vi "Validate Range.vi"(8 "error in (no error)":errorcluster, 11 "Varian Magnet Scan in":refnum<class "Varian Magnet Scan.lvclass">) -> (0 "error out":errorcluster, 3 "Varian Magnet Scan out":refnum<class "Varian Magnet Scan.lvclass">)   [LabVIEW 2009, in "Varian Magnet Scan.lvclass"]
doc: "Coerce the range to be within this Scanner's physical limits."
uses:
  Varian Magnet Scan.lvclass
  Scanner/Scanner.lvclass
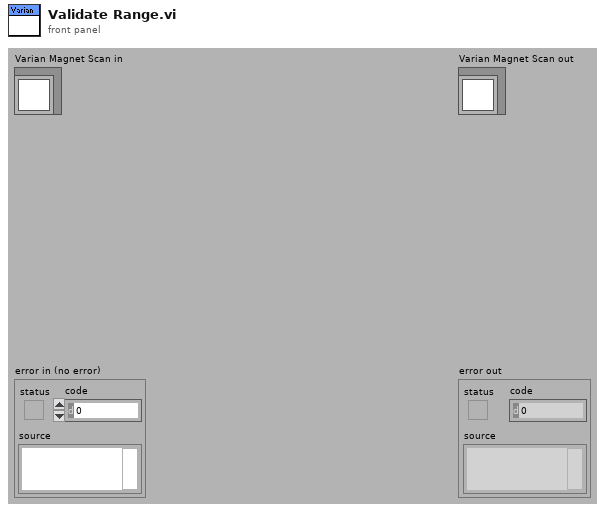
[diagram p1: front panel]
types:
  T1 = typedef "Scanner.lvclass/Range.ctl" = cluster{"xi":dbl, "xf":dbl, "dx":dbl, "Return to...?":bool, "Return to":dbl}
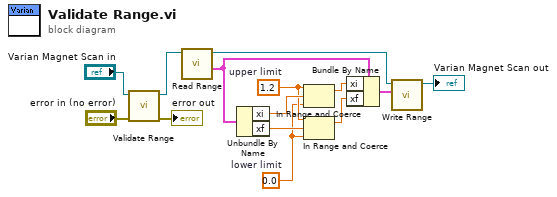
[diagram p0: block diagram]
diagram:
  w8 = 0.0  # lower limit
  w9 = 1.2  # upper limit
  n1 = call-parent "Validate Range.vi"("error in (no error)"="error in (no error)", "Scanner in"="Varian Magnet Scan in") -> ("error out"=→"error out":errorcluster, "Scanner out"=w1:refnum<class "Varian Magnet Scan.lvclass">)  [unwired: 8 in]
  n2 = call-dynamic "Read Range.vi"("Scanner.lvclass in"=w1) -> ("Range"=w6:T1, "Scanner.lvclass out"=w3:refnum<class "Varian Magnet Scan.lvclass">)  [unwired: 5 in, 4 out]
  n3 = Unbundle By Name(w6) -> ("xi"=w11:dbl, "xf"=w10:dbl)
  n4 = In Range and Coerce(upper limit=w9, x=w11, lower limit=w8) -> (coerced(x)=w5:dbl)  [unwired: 1 out]
  n5 = In Range and Coerce(upper limit=w9, x=w10, lower limit=w8) -> (coerced(x)=w4:dbl)  [unwired: 1 out]
  n6 = Bundle By Name(cluster=w6, "xi"=w5, "xf"=w4) -> (w7:T1)
  n7 = call-dynamic "Write Range.vi"("Range"=w7, "Scanner in"=w3) -> ("Scanner out"=→"Varian Magnet Scan out":refnum<class "Varian Magnet Scan.lvclass">)  [unwired: 7 in, 2 out]
